vi "Compare Variant.vi"(2 "Variant 2":variant, 3 "Variant 1":variant) -> (0 "Error?":bool, 1 "Equal?":bool)   [LabVIEW 2015, in "CS++Nanotec.lvlib" / "CS++Nanotec.lvclass"]
doc: "Small utility VI which compares two variant with each other."
uses:
  CS++Nanotec.lvclass
  <vilib>/Utility/Data Type/NI_Data Type.lvlib
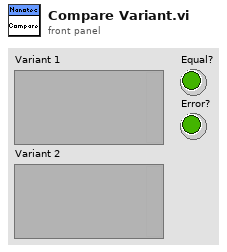
[diagram p1: front panel]
types:
  T1 = typedef "NI_Data Type.lvlib/Data Type.ctl" = enum8{"Invalid Type", "Void", "I8", "I16", "I32", "I64", "U8", "U16", "U32", "U64", "Single Float", "Double Float", "Extended Float", "Single Complex", "Double Complex", "Extended Complex", "Enum U8", "Enum U16", "Enum U32", "Enum U64", "Single Float With Unit", "Double Float With Unit", "Extended Float With Unit", "Single Complex with Unit", "Double Complex with Unit", "Extended Complex with Unit", "Boolean", "String", "Path", "Picture", "Tag", "Array", "Cluster", "Variant", "LV Variant", "Waveform", "Timestamp", "Digital Waveform", "Digital Data", "ExpressData", "Refnum", "External Data", "VI", "Poly VI", "LabVIEW Class Instance", "Fixed Point"}
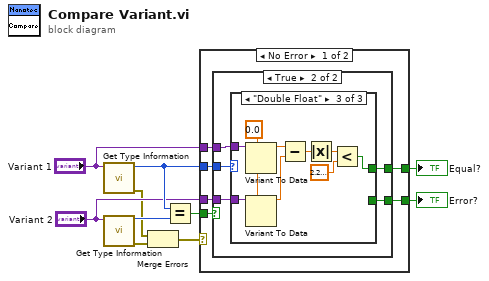
[diagram p0: block diagram]
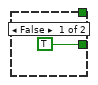
[diagram p2: hidden frame]
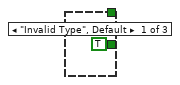
[diagram p3: hidden frame]
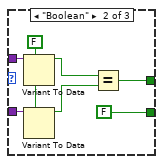
[diagram p4: hidden frame]
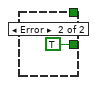
[diagram p5: hidden frame]
diagram:
  n1 = call <vilib>:"Get Type Information.vi"("Variant"="Variant 1") -> ("error out"=w2:errorcluster, "Type"=w9:T1)  [unwired: 6 in, 3 out]
  n2 = call <vilib>:"Get Type Information.vi"("Variant"="Variant 2") -> ("error out"=w3:errorcluster, "Type"=w10:T1)  [unwired: 6 in, 3 out]
  n3 = Merge Errors(w2, w3) -> (w1:errorcluster)
  n4 = Equal?(x=w9, y=w10) -> (x = y?=w8:bool)
  n5 = case shown="No Error" w1 {
    tunnel: w9 -> [w16 _]
    tunnel: w8 -> [w15 _]
    tunnel: "Variant 1" -> [w14 _]
    tunnel: "Variant 2" -> [w13 _]
    tunnel: [w12 _] -> w5
    tunnel: [w11 TRUE] -> w4
    frame No Error {
      n6 = case shown="True" w15 {
        tunnel: w16 -> [_ w22]
        tunnel: w14 -> [_ w21]
        tunnel: w13 -> [_ w20]
        tunnel: [_ w19] -> w12
        tunnel: [TRUE w18] -> w11
        frame False {
        }
        frame True {
          n7 = case shown="\"Double Float\"" w22 {
            tunnel: w21 -> [_ w30 w39]
            tunnel: w20 -> [_ w29 w38]
            tunnel: [_ w25 w32] -> w19
            tunnel: [TRUE FALSE _] -> w18
            frame "Invalid Type", Default {
            }
            frame "Boolean" {
              w28 = FALSE
              n8 = Variant To Data(type=w28, Variant=w30) -> (data=w27:bool)  [unwired: 1 in, 1 out]
              n9 = Variant To Data(type=w28, Variant=w29) -> (data=w26:bool)  [unwired: 1 in, 1 out]
              n10 = Equal?(x=w27, y=w26) -> (x = y?=w25:bool)
            }
            frame "Double Float" {
              w37 = 0.0
              n11 = Variant To Data(type=w37, Variant=w39) -> (data=w36:dbl)  [unwired: 1 in, 1 out]
              n12 = Variant To Data(type=w37, Variant=w38) -> (data=w35:dbl)  [unwired: 1 in, 1 out]
              n13 = Subtract(x=w36, y=w35) -> (x-y=w34:dbl)
              n14 = Absolute Value(x=w34) -> (abs(x)=w33:dbl)
              n15 = Less?(x=w33, y=2.220446049250313e-16) -> (x < y?=w32:bool)
            }
          }
        }
      }
    }
    frame Error {
    }
  }
  "Equal?" <- w5
  "Error?" <- w4
